vi "Pre-Build Action.vi"(6 "Top Level/Always Included VIs":path[](array[path]), 7 "Main Destination Path":path, 9 "Target Name":string, 10 "Build Specification Name":string, 11 "Project Path":path) -> (0 "error out":errorcluster)   [LabVIEW 2020, in "Build VIs.lvlib"]
uses:
  Build VIs.lvlib
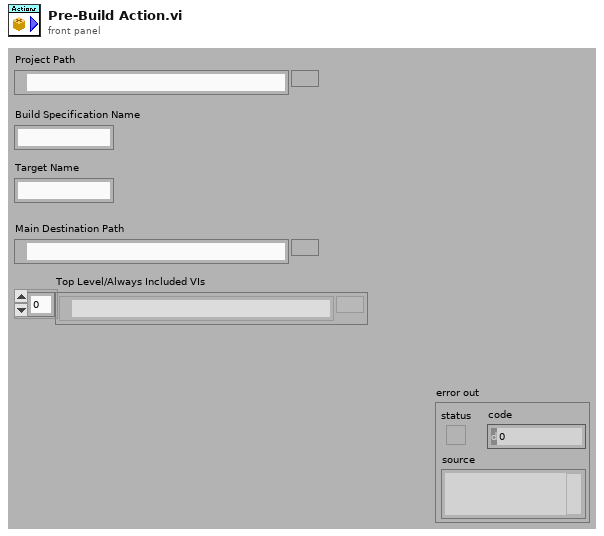
[diagram p1: front panel]
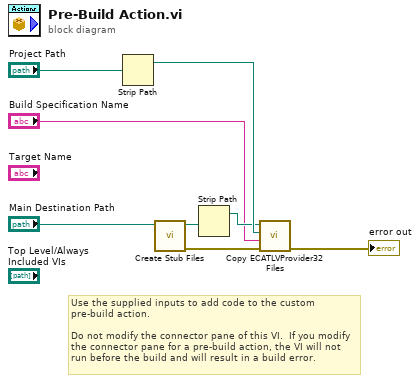
[diagram p0: block diagram]
diagram:
  # "Use the supplied inputs to add code to the custom pre-build action.\n\nDo not modify the connector pane of this VI.  If you modify the connector pane for a pre-build action, the VI will not run before the build and will result in a build error."
  n1 = Strip Path(path="Project Path") -> (stripped path=w5:path)  [unwired: 1 out]
  n2 = call "Create Stub Files.vi"("Main Destination Path"="Main Destination Path") -> ("error out"=w7:errorcluster, "Main Destination Path Out"=w4:path)  [unwired: 9 in]
  n3 = Strip Path(path=w4) -> (stripped path=w3:path)  [unwired: 1 out]
  n4 = call "Copy ECATLVProvider32 Files.vi"("error in"=w7, "Build Specification Name"="Build Specification Name", "Source Path"=w5, "Destination Path"=w3) -> ("error out"=→"error out":errorcluster)  [unwired: 7 in]
